vi "Datalogger_U8_3_byte_Array_to_voltage_current_Rev03.vi"(0 "Nmbr_of_datapoints":dbl=128.0, 1 "Array In":u8[](array[numeric]), 8 "CH1 Shift V":dbl, 15 "AC/DC":bool, 16 "CH0 Shift V":dbl) -> (9 "HEXVAL":string, 11 "CH0 multipler":dbl, 12 "CH1RMS":dbl, 13 "CH2RMS":dbl, 14 "CH1 Vave":dbl, 17 "CH2 Vave":dbl, 19 "CH1 multipler":dbl, 20 "Loop count":dbl, 21 "Voltage":dbl[](graph), 23 "CH1DC":dbl, 24 "Current":dbl[](graph), 25 "mV":dbl, 27 "CH2DC":dbl)   [LabVIEW 2012]
uses:
  <vilib>/measure/madcrms.llb/Basic Averaged DC-RMS for 1 Chan.vi
  <vilib>/measure/NI_MAPro.lvlib
panel:
  out "Array":dbl[](array[numeric])
  out "Numeric 2":dbl
  out "Numeric":dbl
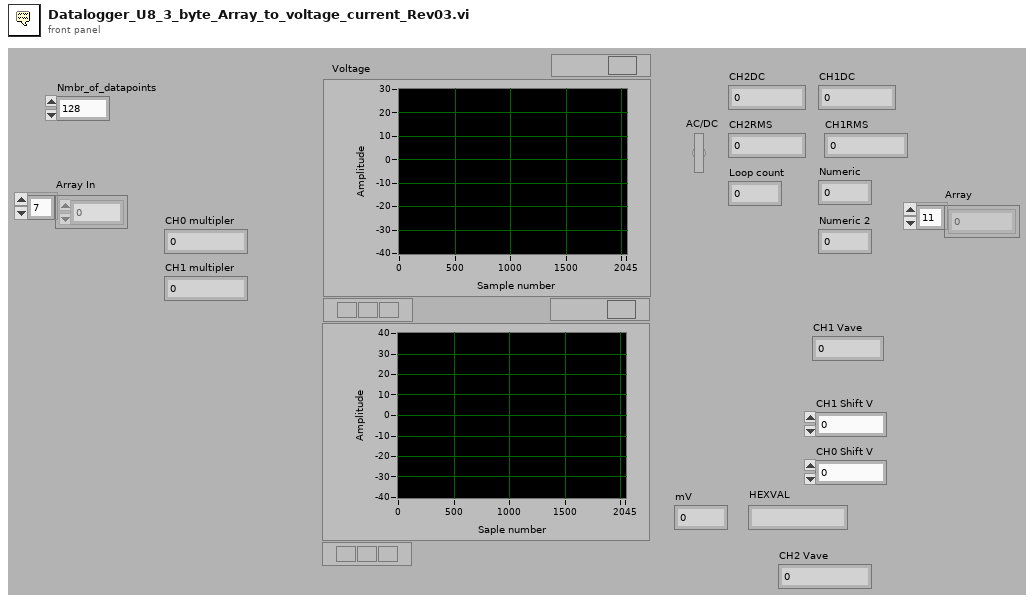
[diagram p1: front panel]
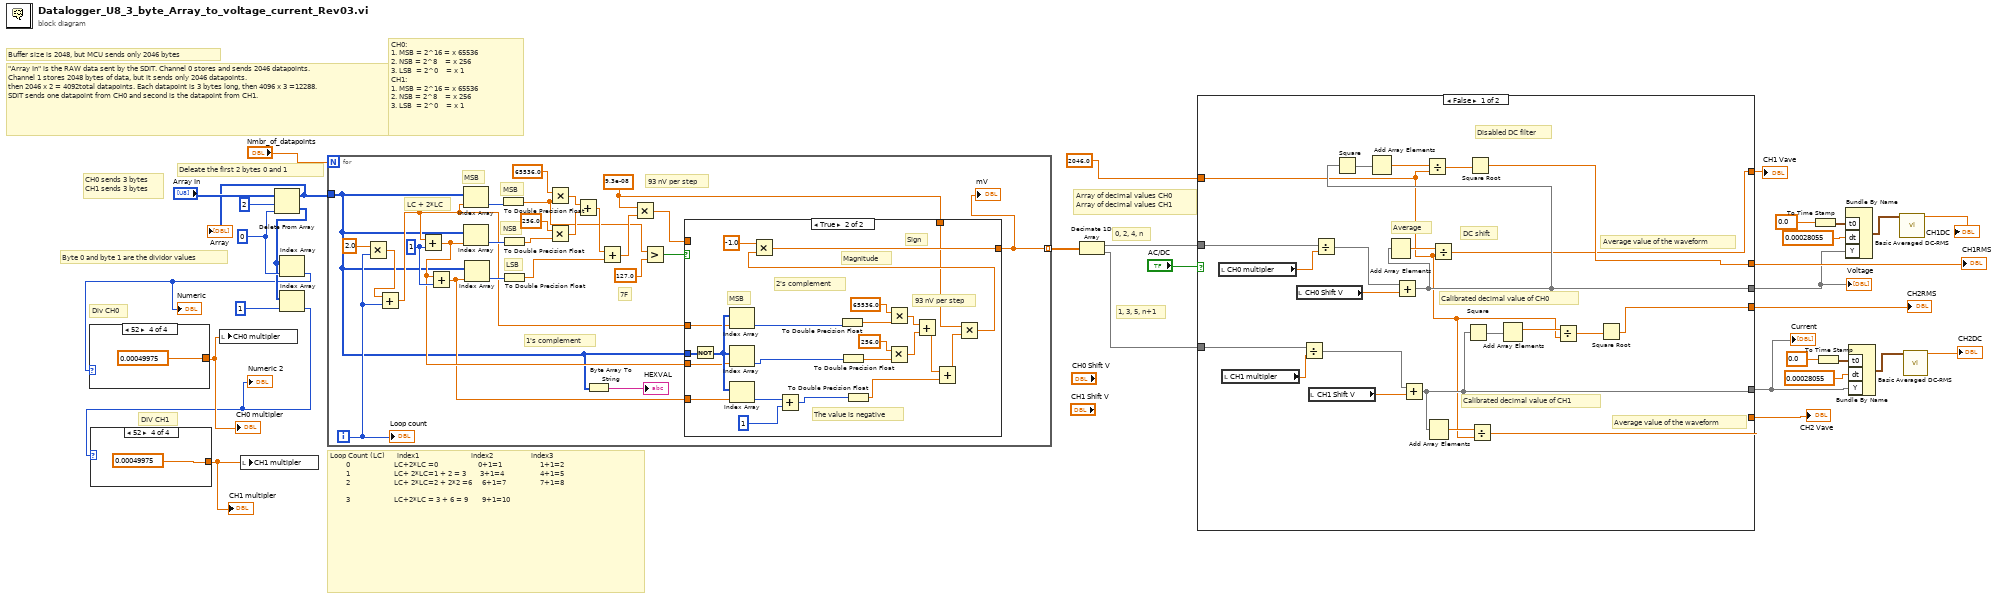
[diagram p0: block diagram]
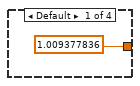
[diagram p2: hidden frame]
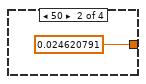
[diagram p3: hidden frame]
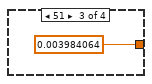
[diagram p4: hidden frame]
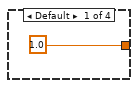
[diagram p5: hidden frame]
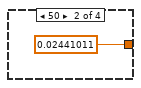
[diagram p6: hidden frame]
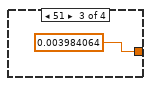
[diagram p7: hidden frame]
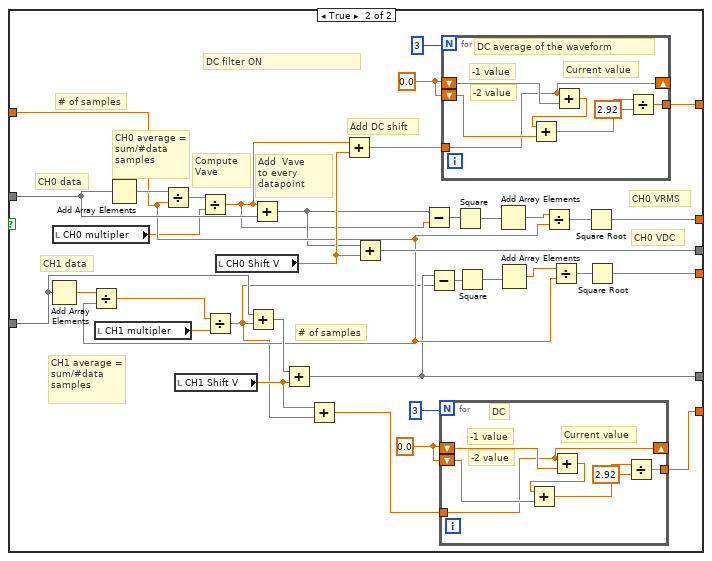
[diagram p8: hidden frame]
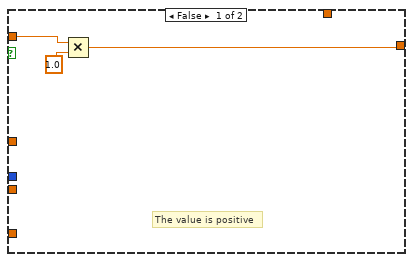
[diagram p9: hidden frame]
diagram:
  w17 = 0
  # "CH0:\n1. MSB = 2^16 = x 65536\n2. NSB = 2^8    = x 256 \n3. LSB  = 2^0    = x 1\nCH1:\n1. MSB = 2^16 = x 65536\n2. NSB = 2^8    = x 256\n3. LSB  = 2^0    = x 1"
  # "Deleate the first 2 bytes 0 and 1"
  # "Buffer size is 2048, but MCU sends only 2046 bytes"
  # "Byte 0 and byte 1 are the dividor values"
  # "DIV CH1"
  # "Div CH0"
  # "\"Array In\" is the RAW data sent by the SDIT. Channel 0 stores and sends 2046 datapoints.\nChannel 1 stores 2048 bytes of data, but it sends only 2046 datapoints.\nthen 2046 x 2 = 4092total datapoints. Each datapoint is 3 bytes long, then 4096 x 3 =12288.\nSDIT sends one datapoint from CH0 and second is the datapoint from CH1."
  # "1, 3, 5, n+1"
  # "0, 2, 4, n"
  # "Array of decimal values CH0\nArray of decimal values CH1"
  # "CH0 sends 3 bytes\nCH1 sends 3 bytes"
  # "Loop Count (LC)      index1                          index2                   index3      \n        0                      LC+2*LC =0                    0+1=1                   1+1=2\n        1                      LC+ 2*LC=1 + 2 = 3       3+1=4                  4+1=5\n        2                      LC+ 2*LC=2 + 2*2 =6     6+1=7                 7+1=8\n\n        3                      LC+2*LC = 3 + 6 = 9       9+1=10"
  n1 = Delete From Array(array="Array In", length=2, index=w17) -> (deleted portion=w15:u8[], array with subset deleted=w1:u8[])
  "Array" <- w1
  n2 = Index Array(array=w15, index=w17) -> (element=w6:u8)
  "Numeric" <- w6
  n3 = case shown="52" w6 {
    tunnel: [1.0 0.02441011 0.003984064 0.00049975] -> w12
    frame Default {
    }
    frame 50 {
    }
    frame 51 {
    }
    frame 52 {
    }
  }
  "CH0 multipler" <- w12
  n4 = local write "CH0 multipler"(w12) -> ()
  n5 = Index Array(array=w15, index=1) -> (element=w5:u8)
  "Numeric 2" <- w5
  n6 = case shown="52" w5 {
    tunnel: [1.009377836 0.024620791 0.003984064 0.00049975] -> w14
    frame Default {
    }
    frame 50 {
    }
    frame 51 {
    }
    frame 52 {
    }
  }
  "CH1 multipler" <- w14
  n7 = local write "CH1 multipler"(w14) -> ()
  n8 = for {
    N: "Nmbr_of_datapoints" -> [_]
    tunnel: w1 -> [w43]
    tunnel: [w42] -> w11 mode=indexing
    i -> [w49]
    w48 = 9.3e-08
    w59 = 1
    # "LC + 2*LC"
    # "7F"
    # "93 nV per step"
    # "LSB"
    # "MSB"
    # "NSB"
    # "1's complement"
    # "MSB"
    n9 = Multiply(x=2.0, y=w49) -> (x*y=w57:dbl)
    n10 = Add(x=w57, y=w49) -> (x+y=w47:dbl)
    n11 = Add(x=w47, y=w59) -> (x+y=w46:dbl)
    n12 = Add(x=w46, y=w59) -> (x+y=w45:dbl)
    n13 = Index Array(array=w43, index=w47) -> (element=w52:u8)
    n14 = Index Array(array=w43, index=w46) -> (element=w51:u8)
    n15 = Index Array(array=w43, index=w45) -> (element=w50:u8)
    n16 = To Double Precision Float(number=w52) -> (double precision float=w53:dbl)
    n17 = To Double Precision Float(number=w51) -> (double precision float=w41:dbl)
    n18 = To Double Precision Float(number=w50) -> (double precision float=w61:dbl)
    n19 = Multiply(x=256.0, y=w41) -> (x*y=w63:dbl)
    n20 = Multiply(x=65536.0, y=w53) -> (x*y=w66:dbl)
    n21 = Add(x=w66, y=w63) -> (x+y=w62:dbl)
    n22 = Byte Array To String(unsigned byte array=w43) -> (string=→"HEXVAL":string)
    n23 = Add(x=w62, y=w61) -> (x+y=w60:dbl)
    n24 = Multiply(x=w48, y=w60) -> (x*y=w56:dbl)
    n25 = Greater?(x=w53, y=127.0) -> (0:w55:bool)
    n26 = case shown="True" w55 {
      tunnel: [w69 w92] -> w42
      tunnel: w56 -> [w68 _]
      tunnel: w43 -> [_ w79]
      tunnel: w47 -> [_ w74]
      tunnel: w46 -> [_ w73]
      tunnel: w45 -> [_ w72]
      tunnel: w48 -> [_ w70]
      frame False {
        # "The value is positive"
        n27 = Multiply(x=w68, y=1.0) -> (x*y=w69:dbl)
      }
      frame True {
        # "The value is negative"
        # "93 nV per step"
        # "Magnitude"
        # "Sign"
        # "2's complement"
        # "MSB"
        n28 = Not(x=w79) -> (.not. x?=w78:u8[])
        n29 = Index Array(array=w78, index=w74) -> (element=w81:u8)
        n30 = Index Array(array=w78, index=w73) -> (element=w80:u8)
        n31 = Index Array(array=w78, index=w72) -> (element=w77:u8)
        n32 = Add(x=w77, y=1) -> (x+y=w75:i32)
        n33 = To Double Precision Float(number=w81) -> (double precision float=w82:dbl)
        n34 = To Double Precision Float(number=w80) -> (double precision float=w88:dbl)
        n35 = To Double Precision Float(number=w75) -> (double precision float=w84:dbl)
        n36 = Multiply(x=256.0, y=w88) -> (x*y=w86:dbl)
        n37 = Multiply(x=65536.0, y=w82) -> (x*y=w90:dbl)
        n38 = Add(x=w90, y=w86) -> (x+y=w85:dbl)
        n39 = Add(x=w85, y=w84) -> (x+y=w83:dbl)
        n40 = Multiply(x=w70, y=w83) -> (x*y=w71:dbl)
        n41 = Multiply(x=-1.0, y=w71) -> (x*y=w92:dbl)
      }
    }
    "mV" <- w42
    "Loop count" <- w49
  }
  n42 = Decimate 1D Array(w11) -> (w10:dbl[], w9:dbl[])
  n43 = case shown="False" "AC/DC" {
    tunnel: w10 -> [w107 w135]
    tunnel: w9 -> [w115 w134]
    tunnel: [w98 w123] -> w2
    tunnel: [w99 w131] -> w4
    tunnel: [w94 w138] -> w31
    tunnel: [w95 w143] -> w30
    tunnel: 2046.0 -> [w96 w126]
    tunnel: [w106 w118] -> w19
    tunnel: [w100 w117] -> w18
    frame False {
      # "Average value of the waveform"
      # "Average value of the waveform"
      # "Disabled DC filter"
      # "Calibrated decimal value of CH1"
      # "Calibrated decimal value of CH0"
      # "DC shift"
      # "Average"
      n44 = local read "CH0 multipler"() -> (w110:dbl)
      n45 = local read "CH1 multipler"() -> (w114:dbl)
      n46 = local read "CH0 Shift V"() -> (w109:dbl)
      n47 = Divide(x=w115, y=w114) -> (x/y=w101:dbl[])
      n48 = local read "CH1 Shift V"() -> (w113:dbl)
      n49 = Divide(x=w107, y=w110) -> (x/y=w112:dbl[])
      n50 = Add(x=w112, y=w109) -> (x+y=w99:dbl[])
      n51 = Square(x=w99) -> (x^2=w108:dbl[])
      n52 = Add Array Elements(numeric array=w108) -> (sum=w93:dbl)
      n53 = Add Array Elements(numeric array=w99) -> (sum=w111:dbl)
      n54 = Add(x=w101, y=w113) -> (x+y=w98:dbl[])
      n55 = Divide(x=w93, y=w96) -> (x/y=w105:dbl)
      n56 = Add Array Elements(numeric array=w98) -> (sum=w97:dbl)
      n57 = Divide(x=w111, y=w96) -> (x/y=w95:dbl)
      n58 = Square(x=w98) -> (x^2=w104:dbl[])
      n59 = Square Root(x=w105) -> (sqrt(x)=w106:dbl)
      n60 = Divide(x=w97, y=w96) -> (x/y=w94:dbl)
      n61 = Add Array Elements(numeric array=w104) -> (sum=w102:dbl)
      n62 = Divide(x=w102, y=w96) -> (x/y=w103:dbl)
      n63 = Square Root(x=w103) -> (sqrt(x)=w100:dbl)
    }
    frame True {
      w140 = 0.0
      w145 = 0.0
      # "DC filter ON"
      # "CH1 average = sum/#data samples"
      # "CH0 VRMS"
      # "CH0 VDC"
      # "Add DC shift"
      # "Compute Vave"
      # "# of samples"
      # "# of samples"
      # "CH1 data"
      # "CH0 data"
      # "Add  Vave\nto every datapoint"
      # "CH0 average = sum/#data samples"
      n64 = Add Array Elements(numeric array=w134) -> (sum=w149:dbl)
      n65 = local read "CH0 multipler"() -> (w116:dbl)
      n66 = Divide(x=w149, y=w126) -> (x/y=w148:dbl)
      n67 = local read "CH1 multipler"() -> (w146:dbl)
      n68 = Add Array Elements(numeric array=w135) -> (sum=w150:dbl)
      n69 = Divide(x=w150, y=w126) -> (x/y=w124:dbl)
      n70 = local read "CH1 Shift V"() -> (w137:dbl)
      n71 = Divide(x=w124, y=w116) -> (x/y=w121:dbl)
      n72 = Divide(x=w148, y=w146) -> (x/y=w122:dbl)
      n73 = local read "CH0 Shift V"() -> (w142:dbl)
      n74 = Add(x=w134, y=w122) -> (x+y=w147:dbl[])
      n75 = Add(x=w121, y=w135) -> (x+y=w125:dbl[])
      n76 = Add(x=w147, y=w137) -> (x+y=w123:dbl[])
      n77 = Add(x=w137, y=w122) -> (x+y=w136:dbl)
      n78 = Add(x=w121, y=w142) -> (x+y=w141:dbl)
      n79 = Add(x=w125, y=w142) -> (x+y=w131:dbl[])
      n80 = Subtract(x=w125, y=w121) -> (x-y=w119:dbl[])
      n81 = Subtract(x=w123, y=w122) -> (x-y=w120:dbl[])
      n82 = for {
        N: 3 -> [_]
        shift-right: [w151] -> _
        shift-left: w140 -> [w157]
        shift-left: w140 -> [w154]
        tunnel: [w152] -> w138
        tunnel: w136 -> [w151]
        # "DC"
        # "-2 value"
        # "-1 value"
        # "Current value"
        n83 = Add(x=w151, y=w157) -> (x+y=w155:dbl)
        n84 = Add(x=w155, y=w154) -> (x+y=w153:dbl)
        n85 = Divide(x=w153, y=2.92) -> (x/y=w152:dbl)
      }
      n86 = for {
        N: 3 -> [_]
        shift-right: [w158] -> _
        shift-left: w145 -> [w164]
        shift-left: w145 -> [w161]
        tunnel: [w159] -> w143
        tunnel: w141 -> [w158]
        # "DC average of the waveform"
        # "-2 value"
        # "-1 value"
        # "Current value"
        n87 = Add(x=w158, y=w164) -> (x+y=w162:dbl)
        n88 = Add(x=w162, y=w161) -> (x+y=w160:dbl)
        n89 = Divide(x=w160, y=2.92) -> (x/y=w159:dbl)
      }
      n90 = Square(x=w119) -> (x^2=w130:dbl[])
      n91 = Square(x=w120) -> (x^2=w127:dbl[])
      n92 = Add Array Elements(numeric array=w130) -> (sum=w132:dbl)
      n93 = Add Array Elements(numeric array=w127) -> (sum=w128:dbl)
      n94 = Divide(x=w132, y=w126) -> (x/y=w133:dbl)
      n95 = Divide(x=w128, y=w126) -> (x/y=w129:dbl)
      n96 = Square Root(x=w133) -> (sqrt(x)=w118:dbl)
      n97 = Square Root(x=w129) -> (sqrt(x)=w117:dbl)
    }
  }
  "Current" <- w2
  "Voltage" <- w4
  "CH2 Vave" <- w31
  "CH1 Vave" <- w30
  "CH1RMS" <- w19
  "CH2RMS" <- w18
  n98 = To Time Stamp(1:0.0 ("t0")) -> (0:w28:timestamp)
  n99 = To Time Stamp(1:0.0 ("t0")) -> (0:w24:timestamp)
  n100 = Bundle By Name("t0"=w28, "dt"=0.00028055, "Y"=w4) -> (w29:waveform(dbl))  [unwired: 1 in]
  n101 = Bundle By Name("t0"=w24, "dt"=0.00028055, "Y"=w2) -> (w25:waveform(dbl))  [unwired: 1 in]
  n102 = call-poly <vilib>:"Basic Averaged DC-RMS.vi"("signal in"=w29) -> ("DC value"=→"CH1DC":dbl)  [unwired: 7 in, 3 out]
  n103 = call-poly <vilib>:"Basic Averaged DC-RMS.vi"("signal in"=w25) -> ("DC value"=→"CH2DC":dbl)  [unwired: 7 in, 3 out]
